vi "RhinoTrackCode.vi"(0 "Y Driver Control":dbl, 1 "Manual Aim Mode":bool, 2 "Auto aimer":bool, 5 "X Driver Control":dbl, 9 "Shooter Y":dbl, 11 "Shooter X":dbl, 12 "Distance":dbl) -> (3 "Driver Control":bool, 4 "Left Driver 1":dbl, 6 "Left Driver 2":dbl, 8 "Right Driver 1":dbl, 10 "Right Driver 2":dbl, 13 "Autoaim?":bool, 14 "Aiming stuff":T1, 15 "Shooter Y Motion":dbl)   [LabVIEW 2015]
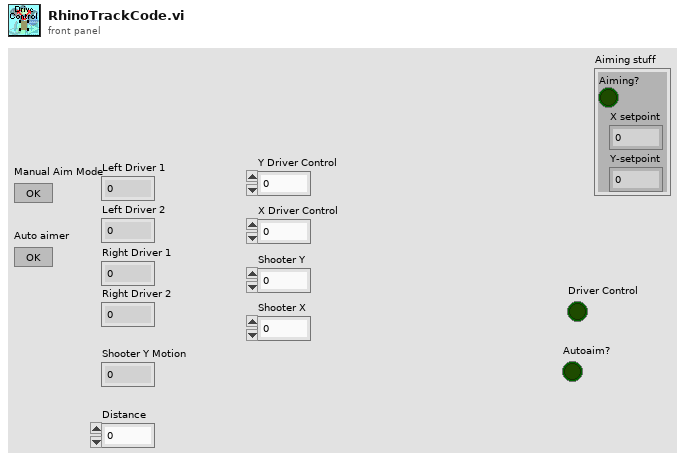
[diagram p1: front panel]
types:
  T1 = cluster{"Aiming?":bool, "X setpoint":dbl, "Y-setpoint":dbl}
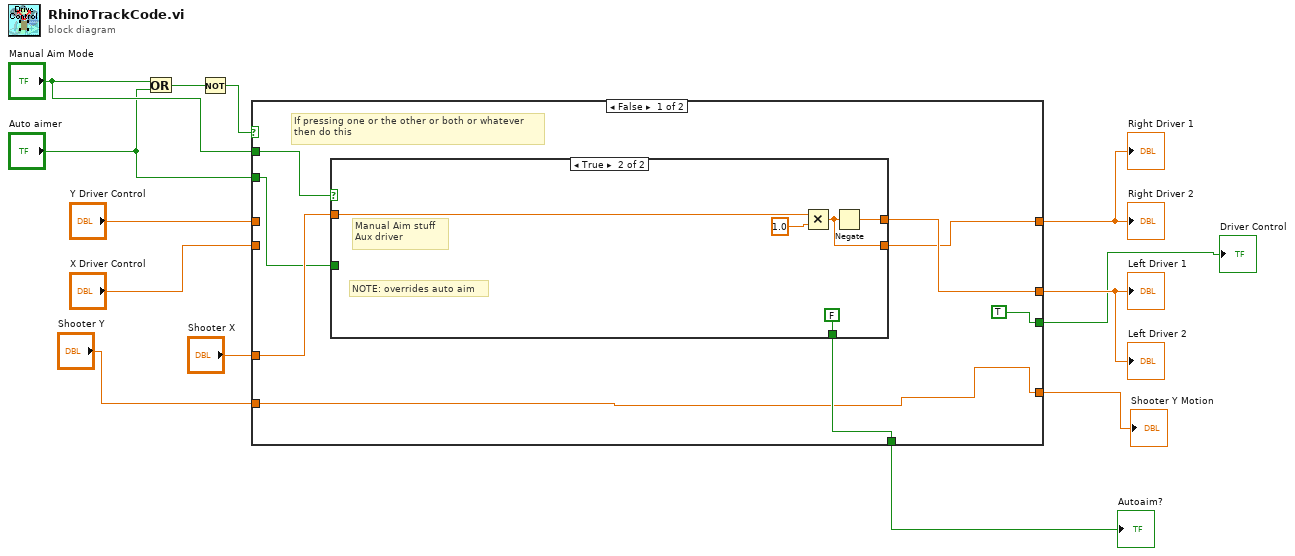
[diagram p0: block diagram]
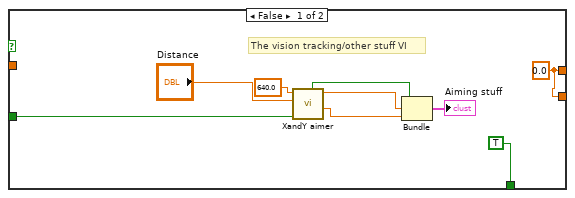
[diagram p2: hidden frame]
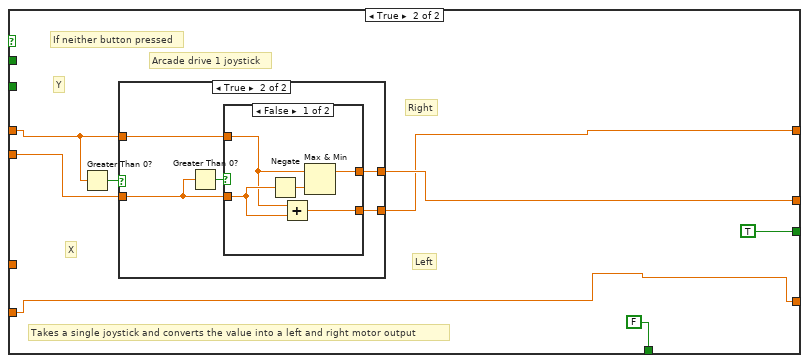
[diagram p3: hidden frame]
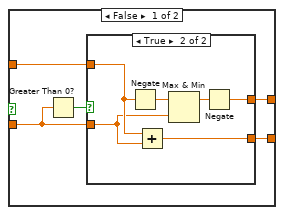
[diagram p4: hidden frame]
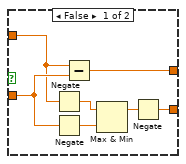
[diagram p5: hidden frame]
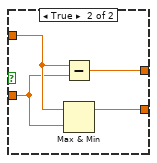
[diagram p6: hidden frame]
diagram:
  n1 = Or(x="Manual Aim Mode", y="Auto aimer") -> (x .or. y?=w7:bool)
  n2 = Not(x=w7) -> (.not. x?=w6:bool)
  n3 = case shown="False" w6 {
    tunnel: "Y Driver Control" -> [_ w40]
    tunnel: "X Driver Control" -> [_ w39]
    tunnel: [w19 w41] -> w11
    tunnel: [w20 w42] -> w10
    tunnel: "Shooter X" -> [w21 _]
    tunnel: "Manual Aim Mode" -> [w18 _]
    tunnel: [w15 w37] -> w8
    tunnel: "Auto aimer" -> [w17 _]
    tunnel: [w16 FALSE] -> w3
    tunnel: "Shooter Y" -> [w15 w37]
    tunnel: [TRUE TRUE] -> w1
    frame False {
      # "If pressing one or the other or both or whatever\nthen do this"
      n4 = case shown="True" w18 {
        tunnel: w21 -> [_ w33]
        tunnel: [w27 w35] -> w20
        tunnel: [w27 w32] -> w19
        tunnel: w17 -> [w30 _]
        tunnel: [TRUE FALSE] -> w16
        frame False {
          w27 = 0.0
          # "The vision tracking/other stuff VI"
          n5 = call "XandY aimer.vi"("Aiming?"=w30, "Distance"="Distance", "Image width"=640.0) -> ("Y-setpoint"=w25:dbl, "X setpoint"=w24:dbl, "Aiming?"=w26:bool)  [unwired: 5 in, 1 out]
          n6 = Bundle("Aiming?"=w26, "X setpoint"=w24, "Y-setpoint"=w25) -> (→"Aiming stuff":T1)  [unwired: 1 in]
        }
        frame True {
          # "NOTE: overrides auto aim"
          # "Manual Aim stuff\nAux driver"
          n7 = Multiply(x=w33, y=1.0) -> (x*y=w32:dbl)
          n8 = Negate(x=w32) -> (-x=w35:dbl)
        }
      }
    }
    frame True {
      # "Takes a single joystick and converts the value into a left and right motor output"
      # "If neither button pressed"
      # "Arcade drive 1 joystick"
      # "X"
      # "Y"
      # "Right"
      # "Left"
      n9 = Greater Than 0?(x=w40) -> (x > 0?=w43:bool)
      n10 = case shown="True" w43 {
        tunnel: w39 -> [w47 w65]
        tunnel: w40 -> [w46 w64]
        tunnel: [w45 w63] -> w42
        tunnel: [w44 w62] -> w41
        frame False {
          n11 = Greater Than 0?(x=w47) -> (x > 0?=w48:bool)
          n12 = case shown="True" w48 {
            tunnel: w47 -> [w55 w57]
            tunnel: w46 -> [w53 w58]
            tunnel: [w49 w59] -> w45
            tunnel: [w50 w56] -> w44
            frame False {
              n13 = Negate(x=w53) -> (-x=w54:dbl)
              n14 = Negate(x=w55) -> (-x=w52:dbl)
              n15 = Subtract(x=w53, y=w55) -> (x-y=w49:dbl)
              n16 = Max & Min(x=w54, y=w52) -> (max(x,y)=w51:dbl)  [unwired: 1 out]
              n17 = Negate(x=w51) -> (-x=w50:dbl)
            }
            frame True {
              n18 = Negate(x=w58) -> (-x=w61:dbl)
              n19 = Add(x=w58, y=w57) -> (x+y=w56:dbl)
              n20 = Max & Min(x=w61, y=w57) -> (max(x,y)=w60:dbl)  [unwired: 1 out]
              n21 = Negate(x=w60) -> (-x=w59:dbl)
            }
          }
        }
        frame True {
          n22 = Greater Than 0?(x=w65) -> (x > 0?=w66:bool)
          n23 = case shown="False" w66 {
            tunnel: w65 -> [w71 w73]
            tunnel: w64 -> [w68 w74]
            tunnel: [w69 w72] -> w63
            tunnel: [w67 w75] -> w62
            frame False {
              n24 = Negate(x=w71) -> (-x=w70:dbl)
              n25 = Add(x=w68, y=w71) -> (x+y=w67:dbl)
              n26 = Max & Min(x=w68, y=w70) -> (max(x,y)=w69:dbl)  [unwired: 1 out]
            }
            frame True {
              n27 = Subtract(x=w74, y=w73) -> (x-y=w72:dbl)
              n28 = Max & Min(x=w74, y=w73) -> (max(x,y)=w75:dbl)  [unwired: 1 out]
            }
          }
        }
      }
    }
  }
  "Left Driver 1" <- w10
  "Left Driver 2" <- w10
  "Right Driver 2" <- w11
  "Right Driver 1" <- w11
  "Shooter Y Motion" <- w8
  "Autoaim?" <- w3
  "Driver Control" <- w1
